vi "Convert to Client Init Type.vi"(11 "initialize and close session behavior":T1) -> (3 "initialize_and_close_session_behavior":T2)   [LabVIEW 2021, in "SimpleSwitchConnect.lvlib"]
uses:
  SimpleSwitchConnect.lvlib
  <vilib>/Plug-In SDKs/Clients/Session Management V1/Session Reservation/Initialize and Close Session Behavior.ctl
  <vilib>/Plug-In SDKs/Sessions/Instrument/ISession Factory/Initialize and Close Session Behavior.ctl
  <vilib>/Plug-In SDKs/Clients/Session Management V1/Session Reservation/Session Reservation.lvclass
  <vilib>/Plug-In SDKs/Sessions/Instrument/ISession Factory/ISession Factory.lvclass
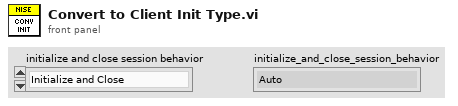
[diagram p1: front panel]
types:
  T1 = typedef "NI Session Management Instrument.lvlib/ISession Factory.lvclass/Initialize and Close Session Behavior.ctl" = enum16{"Initialize and Close", "Attach and Detach", "Initialize and Detach", "Attach and Close"}
  T2 = typedef "NI Session Management V1 Client.lvlib/Session Reservation.lvclass/Initialize and Close Session Behavior.ctl" = enum16{"Auto", "Initialize and Close", "Attach and Detach", "Initialize and Detach", "Attach and Close"}
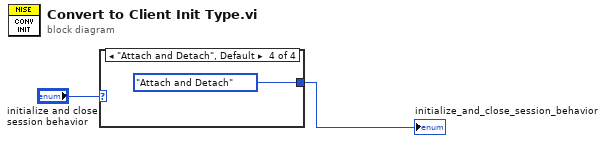
[diagram p0: block diagram]
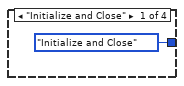
[diagram p2: hidden frame]
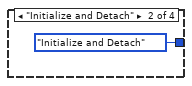
[diagram p3: hidden frame]
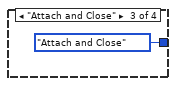
[diagram p4: hidden frame]
diagram:
  n1 = case shown="\"Attach and Detach\", Default" "initialize and close session behavior" {
    tunnel: [Initialize_and_Close_Session_Behavior."Initialize and Close" ("initialize_and_close_session_behavior") Initialize_and_Close_Session_Behavior."Initialize and Detach" ("initialize_and_close_session_behavior") Initialize_and_Close_Session_Behavior."Attach and Close" ("initialize_and_close_session_behavior") Initialize_and_Close_Session_Behavior."Attach and Detach" ("initialize_and_close_session_behavior")] -> w2
    frame "Initialize and Close" {
    }
    frame "Initialize and Detach" {
    }
    frame "Attach and Close" {
    }
    frame "Attach and Detach", Default {
    }
  }
  "initialize_and_close_session_behavior" <- w2
